vi "Acquisition_Dialog.vi"(1 "Scan Parameters file path":path, 11 "error in":errorcluster) -> (3 "Replay settings out":T17={"Sampling Rate"=0.0, "Samples in replay"=0, "Replay Start Time"=1000.0, "Replay Stop Time"=0.003} {"Replay Stop Time" format="%.3p"; "Replay Start Time" format="%.3p"}, 4 "Acquisition Unit Out":i32, 6 "Acquire Defn Out":T1={"Acquire Mode"=enum."stop", "Acquisition mode"=enum."Sampled", "Acquirer"=enum."Cleverscope", "Transfer Chans"=enum."Chan A+B", "A max scale"=5.0, "A min scale"=-5.0, "B max scale"=5.0, "B min scale"=-5.0, "A Probe"=enum."x1", "B Probe"=enum."x1", "A Coupling"=enum."DC", "B Coupling"=enum."DC", "A Bandwidth"=1, "B Bandwidth"=1, "Trigger Source"=enum."Chan A", "Trigger Amplitude"=0.0, "A Trigger Amplitude"=0.0, "B Trigger Amplitude"=0.0, "Trigger Filter"=enum."None", "Trig Slope"=FALSE, "Trigger Holdoff"=0.0, "Dig Pattern Rqd"=FALSE, "Dig Pattern"=0, "Ext Trig Threshold"=0.0, "Dig Input Threshold"=0.0, "Start Time"=-0.003, "Stop Time"=0.003, "Pre Trig Time"=0.003, "Port"=enum."Port 1", "Num divisions"=6, "Num seq frames"=1, "Num Buffers"=2, "Sig Gen Freq"=1000.0, "Sig Gen Amp"=1.0, "Sig Gen Offset"=0.0, "Sig Gen Waveform"=enum."sine", "Sig Gen Sweep"=enum."Log", "Sig Gen Func"=enum."Standard", "Sig Gen Freq 2"=1000.0, "Sig Gen Phase"=180.0, "Trig 2 Function"=enum."None", "Min Trigger Period"=1e-08, "Max trigger Period"=0.0001, "Trigger count"=1, "Trig 2 Slope"=FALSE, "Trig 2 Source Chan"=enum."Chan A", "Trig 2 Level"=0.0, "Dig Pattern 2 Rqd"=FALSE, "Dig Pattern 2"=0, "Trigger 2 Source"=enum."Trigger 1 inverted", "Waveform Averages"=0, "Value changed"=0, "Freq Span"=0.0, "Freq Res"=0.0, "Duration"=0.0, "Resolution"=0.0, "Link Port"=enum."Debug", "Ext Sample Clock"=FALSE, "F Spare 2"=FALSE, "F Spare 3"=FALSE, "F Spare 4"=FALSE, "Sampler Resolution"=enum."10 bit", "Intf Source"=enum."USB", "Update Rate"=enum."20 Frame/sec", "Transfer Size"=enum."Normal", "Sig Gen Freq Step"=0.0, "TCP Adr"=0, "TCP port"=0, "CAU Ser Num Hi"=0, "CAU Ser Num Lo"=0, "Function Number"=0.0, "Function Parameter"=0.0, "Function Result"=0.0, "Link Start"=0, "Link Timebase"=0, "Link Timer"=0, "Link Setup"=0, "Spare 1"=0.0, "Spare 2"=0.0, "Spare 3"=0.0, "Spare 4"=0.0} {"Function Result" format="%#.6p"; "Function Parameter" format="%#.6p"; "Function Number" format="%#.6p"; "TCP Adr" format="%08x"; "Sig Gen Freq Step" format="%.2f"; "Sig Gen Phase" format="%.2f"; "Sig Gen Freq 2" format="%.2f"; "Resolution" format="%#.6p"; "Duration" format="%#.6p"; "Freq Res" format="%#.6p"; "Freq Span" format="%#.6p"; "Dig Pattern 2" format="%.0x"; "Trig 2 Level" step=0.001 format="%#.6p"; "Trigger count" step=1; "Max trigger Period" min=1e-08 max=42.9 step=0.01 format="%#.6p"; "Min Trigger Period" min=1e-08 max=42.9 step=0.01 format="%#_6p"; "Sig Gen Offset" format="%.2f"; "Sig Gen Amp" format="%.2f"; "Sig Gen Freq" format="%.2f"; "B Trigger Amplitude" format="%.1p"; "A Trigger Amplitude" format="%.1p"; "B Bandwidth" format="%x"; "A Bandwidth" format="%x"; "B min scale" format="%.2p"; "B max scale" format="%.2p"; "A min scale" format="%.2p"; "A max scale" format="%.2p"; "Trigger Holdoff" format="%.1p"; "Dig Input Threshold" format="%.2f"; "Ext Trig Threshold" format="%.2f"; "Dig Pattern" format="%.0x"; "Pre Trig Time" format="%.3p"; "Start Time" format="%.2p"; "Trigger Amplitude" format="%.1p"; "Stop Time" format="%.2p"}, 8 "Cancelled?":bool, 15 "error out":errorcluster)   [LabVIEW 2009]
uses:
  libraries/Cscope control driver.llb/Acquire Event type.ctl
  libraries/Cscope control driver.llb/Acquire capture type.ctl
  libraries/Cscope control driver.llb/Acquire capture method.ctl
  libraries/Cscope control driver.llb/Acquirer type.ctl
  libraries/Cscope control driver.llb/Input Range.ctl
  libraries/Cscope control driver.llb/Input Coupling.ctl
  libraries/Cscope control driver.llb/Input Bandwidth.ctl
  libraries/Cscope control driver.llb/USB channel.ctl
  libraries/Cscope control driver.llb/Trigger Filter.ctl
  libraries/Cscope control driver.llb/Cscope waveform type.ctl
  libraries/Cscope control driver.llb/Trigger Period.ctl
  libraries/Cscope control driver.llb/Trigger channel.ctl
  libraries/Cscope control driver.llb/Link port types.ctl
  libraries/Cscope control driver.llb/Acquirer resolution.ctl
  libraries/Cscope control driver.llb/Intf source.ctl
  libraries/Cscope control driver.llb/Acquire transfer size.ctl
  typedefs/Cscope/ReplaySettings.ctl
  libraries/Cscope control driver.llb/Digital Pattern.ctl
  libraries/Cscope control driver.llb/Digital And Or.ctl
  libraries/Cscope control driver.llb/Digital And Or option.ctl
  libraries/Cscope control driver.llb/Digital Masks.ctl
  libraries/Cscope control driver.llb/Dig Control.ctl
  typedefs/Cscope/Connection Settings.ctl
  typedefs/Cscope/TriggerDefn.ctl
  typedefs/AcquisitionDialog_States.ctl
panel:
  in  "Acquire Defn":T1={"Acquire Mode"=enum."stop", "Acquisition mode"=enum."Sampled", "Acquirer"=enum."Cleverscope", "Transfer Chans"=enum."Chan A+B", "A max scale"=5.0, "A min scale"=-5.0, "B max scale"=5.0, "B min scale"=-5.0, "A Probe"=enum."x1", "B Probe"=enum."x1", "A Coupling"=enum."DC", "B Coupling"=enum."DC", "A Bandwidth"=1, "B Bandwidth"=1, "Trigger Source"=enum."Chan A", "Trigger Amplitude"=0.0, "A Trigger Amplitude"=0.0, "B Trigger Amplitude"=0.0, "Trigger Filter"=enum."None", "Trig Slope"=FALSE, "Trigger Holdoff"=0.0, "Dig Pattern Rqd"=FALSE, "Dig Pattern"=0, "Ext Trig Threshold"=0.0, "Dig Input Threshold"=0.0, "Start Time"=-0.003, "Stop Time"=0.003, "Pre Trig Time"=0.003, "Port"=enum."Port 1", "Num divisions"=6, "Num seq frames"=1, "Num Buffers"=2, "Sig Gen Freq"=1000.0, "Sig Gen Amp"=1.0, "Sig Gen Offset"=0.0, "Sig Gen Waveform"=enum."sine", "Sig Gen Sweep"=enum."Log", "Sig Gen Func"=enum."Standard", "Sig Gen Freq 2"=1000.0, "Sig Gen Phase"=180.0, "Trig 2 Function"=enum."None", "Min Trigger Period"=1e-08, "Max trigger Period"=0.0001, "Trigger count"=1, "Trig 2 Slope"=FALSE, "Trig 2 Source Chan"=enum."Chan A", "Trig 2 Level"=0.0, "Dig Pattern 2 Rqd"=FALSE, "Dig Pattern 2"=0, "Trigger 2 Source"=enum."Trigger 1 inverted", "Waveform Averages"=0, "Value changed"=0, "Freq Span"=0.0, "Freq Res"=0.0, "Duration"=0.0, "Resolution"=0.0, "Link Port"=enum."Debug", "Ext Sample Clock"=FALSE, "F Spare 2"=FALSE, "F Spare 3"=FALSE, "F Spare 4"=FALSE, "Sampler Resolution"=enum."10 bit", "Intf Source"=enum."USB", "Update Rate"=enum."20 Frame/sec", "Transfer Size"=enum."Normal", "Sig Gen Freq Step"=0.0, "TCP Adr"=0, "TCP port"=0, "CAU Ser Num Hi"=0, "CAU Ser Num Lo"=0, "Function Number"=0.0, "Function Parameter"=0.0, "Function Result"=0.0, "Link Start"=0, "Link Timebase"=0, "Link Timer"=0, "Link Setup"=0, "Spare 1"=0.0, "Spare 2"=0.0, "Spare 3"=0.0, "Spare 4"=0.0} {"Function Result" format="%#.6p"; "Function Parameter" format="%#.6p"; "Function Number" format="%#.6p"; "TCP Adr" format="%08x"; "Sig Gen Freq Step" format="%.2f"; "Sig Gen Phase" format="%.2f"; "Sig Gen Freq 2" format="%.2f"; "Resolution" format="%#.6p"; "Duration" format="%#.6p"; "Freq Res" format="%#.6p"; "Freq Span" format="%#.6p"; "Dig Pattern 2" format="%.0x"; "Trig 2 Level" step=0.001 format="%#.6p"; "Trigger count" step=1; "Max trigger Period" min=1e-08 max=42.9 step=0.01 format="%#.6p"; "Min Trigger Period" min=1e-08 max=42.9 step=0.01 format="%#_6p"; "Sig Gen Offset" format="%.2f"; "Sig Gen Amp" format="%.2f"; "Sig Gen Freq" format="%.2f"; "B Trigger Amplitude" format="%.1p"; "A Trigger Amplitude" format="%.1p"; "B Bandwidth" format="%x"; "A Bandwidth" format="%x"; "B min scale" format="%.2p"; "B max scale" format="%.2p"; "A min scale" format="%.2p"; "A max scale" format="%.2p"; "Trigger Holdoff" format="%.1p"; "Dig Input Threshold" format="%.2f"; "Ext Trig Threshold" format="%.2f"; "Dig Pattern" format="%.0x"; "Pre Trig Time" format="%.3p"; "Start Time" format="%.2p"; "Trigger Amplitude" format="%.1p"; "Stop Time" format="%.2p"}
  in  "Tab Control":T18(tab)
  in  "Trigger 1 Definition":T24={"Source"=enum."Chan A", "Level"=0.0, "Slope"=FALSE, "Dig Pattern"={"Digital Or Mask"={"1"=FALSE, "2"=FALSE, "3"=FALSE, "4"=FALSE, "5"=FALSE, "6"=FALSE, "7"=FALSE, "8"=FALSE}, "Digital Masks"={"8"=enum."C", "7"=enum."C", "6"=enum."C", "5"=enum."C", "4"=enum."C", "3"=enum."C", "2"=enum."C", "1"=enum."Ý"}}, "Digital \nPattern"=FALSE, "Filter"=enum."None"} {"Level" step=0.001 format="%#.6p"}
  in  "Channel Settings":T25={"A max scale"=1.0, "A min scale"=-1.0, "B max scale"=5.0, "B min scale"=-5.0, "A Probe"=enum."x1", "B Probe"=enum."x1", "A Coupling"=enum."DC", "B Coupling"=enum."DC", "A Filter"=FALSE, "B Filter"=FALSE} {"B min scale" format="%.2p"; "B max scale" format="%.2p"; "A min scale" format="%.2p"; "A max scale" format="%.2p"}
  in  "Force Select":T26(radio)
  in  "Replay Settings":T17={"Sampling Rate"=0.0, "Samples in replay"=0, "Replay Start Time"=1000.0, "Replay Stop Time"=0.003} {"Replay Stop Time" format="%.3p"; "Replay Start Time" format="%.3p"}
  in  "Acquisition Unit":i32
  in  "Acquisition Settings":T27={"Acquire Mode"=enum."single", "Acquisition mode"=enum."Sampled", "Onboard\nWaveform Averages"=0, "Number of Averages"=1, "Sampler Resolution"=enum."12 Bit", "Ext Sample Clock"=FALSE} {"Onboard\nWaveform Averages" scale=4.0..128.0; "Number of Averages" max=2999}
  in  "Sync Signal Settings":T28={"Pulse Repitition Interval"=333.33, "Amplitude"=2.0}
  in  "Filtering":T29 {"Pre-Filter A" items=["None", "20 MHz filter"]; "Pre-Filter B" items=["None", "20 MHz filter"]; "Moving Average" items=["40 ns"=1, "80 ns"=2, "160 ns"=3, "320 ns"=4, "640 ns"=5, "1.28 us"=6]}
  in  "Trigger 2 Source":enum16{"Trigger 1 inverted", "Trig 2 Defn"}(ring)
  in  "Trigger 2 Definition":T30={"Source"=enum."Chan A", "Level"=0.0, "Slope"=FALSE, "Dig Pattern"={"Digital Or Mask"={"1"=FALSE, "2"=FALSE, "3"=FALSE, "4"=FALSE, "5"=FALSE, "6"=FALSE, "7"=FALSE, "8"=FALSE}, "Digital Masks"={"8"=enum."C", "7"=enum."C", "6"=enum."C", "5"=enum."C", "4"=enum."C", "3"=enum."C", "2"=enum."C", "1"=enum."Ý"}}, "Digital \nPattern"=FALSE} {"Level" step=0.001 format="%#.6p"}
  in  "Trig 1~2":T31={"Trig 2 Function"=enum."None", "Min Trigger Period"=1e-08, "Max trigger Period"=0.0001, "Trigger count"=1} {"Trigger count" step=1; "Max trigger Period" min=1e-08 max=42.9 step=0.01 format="%#.6p"; "Min Trigger Period" min=1e-08 max=42.9 step=0.01 format="%#_6p"}
  in  "Connection Settings":T32
  in  "Cancel":bool
  in  "OK":bool
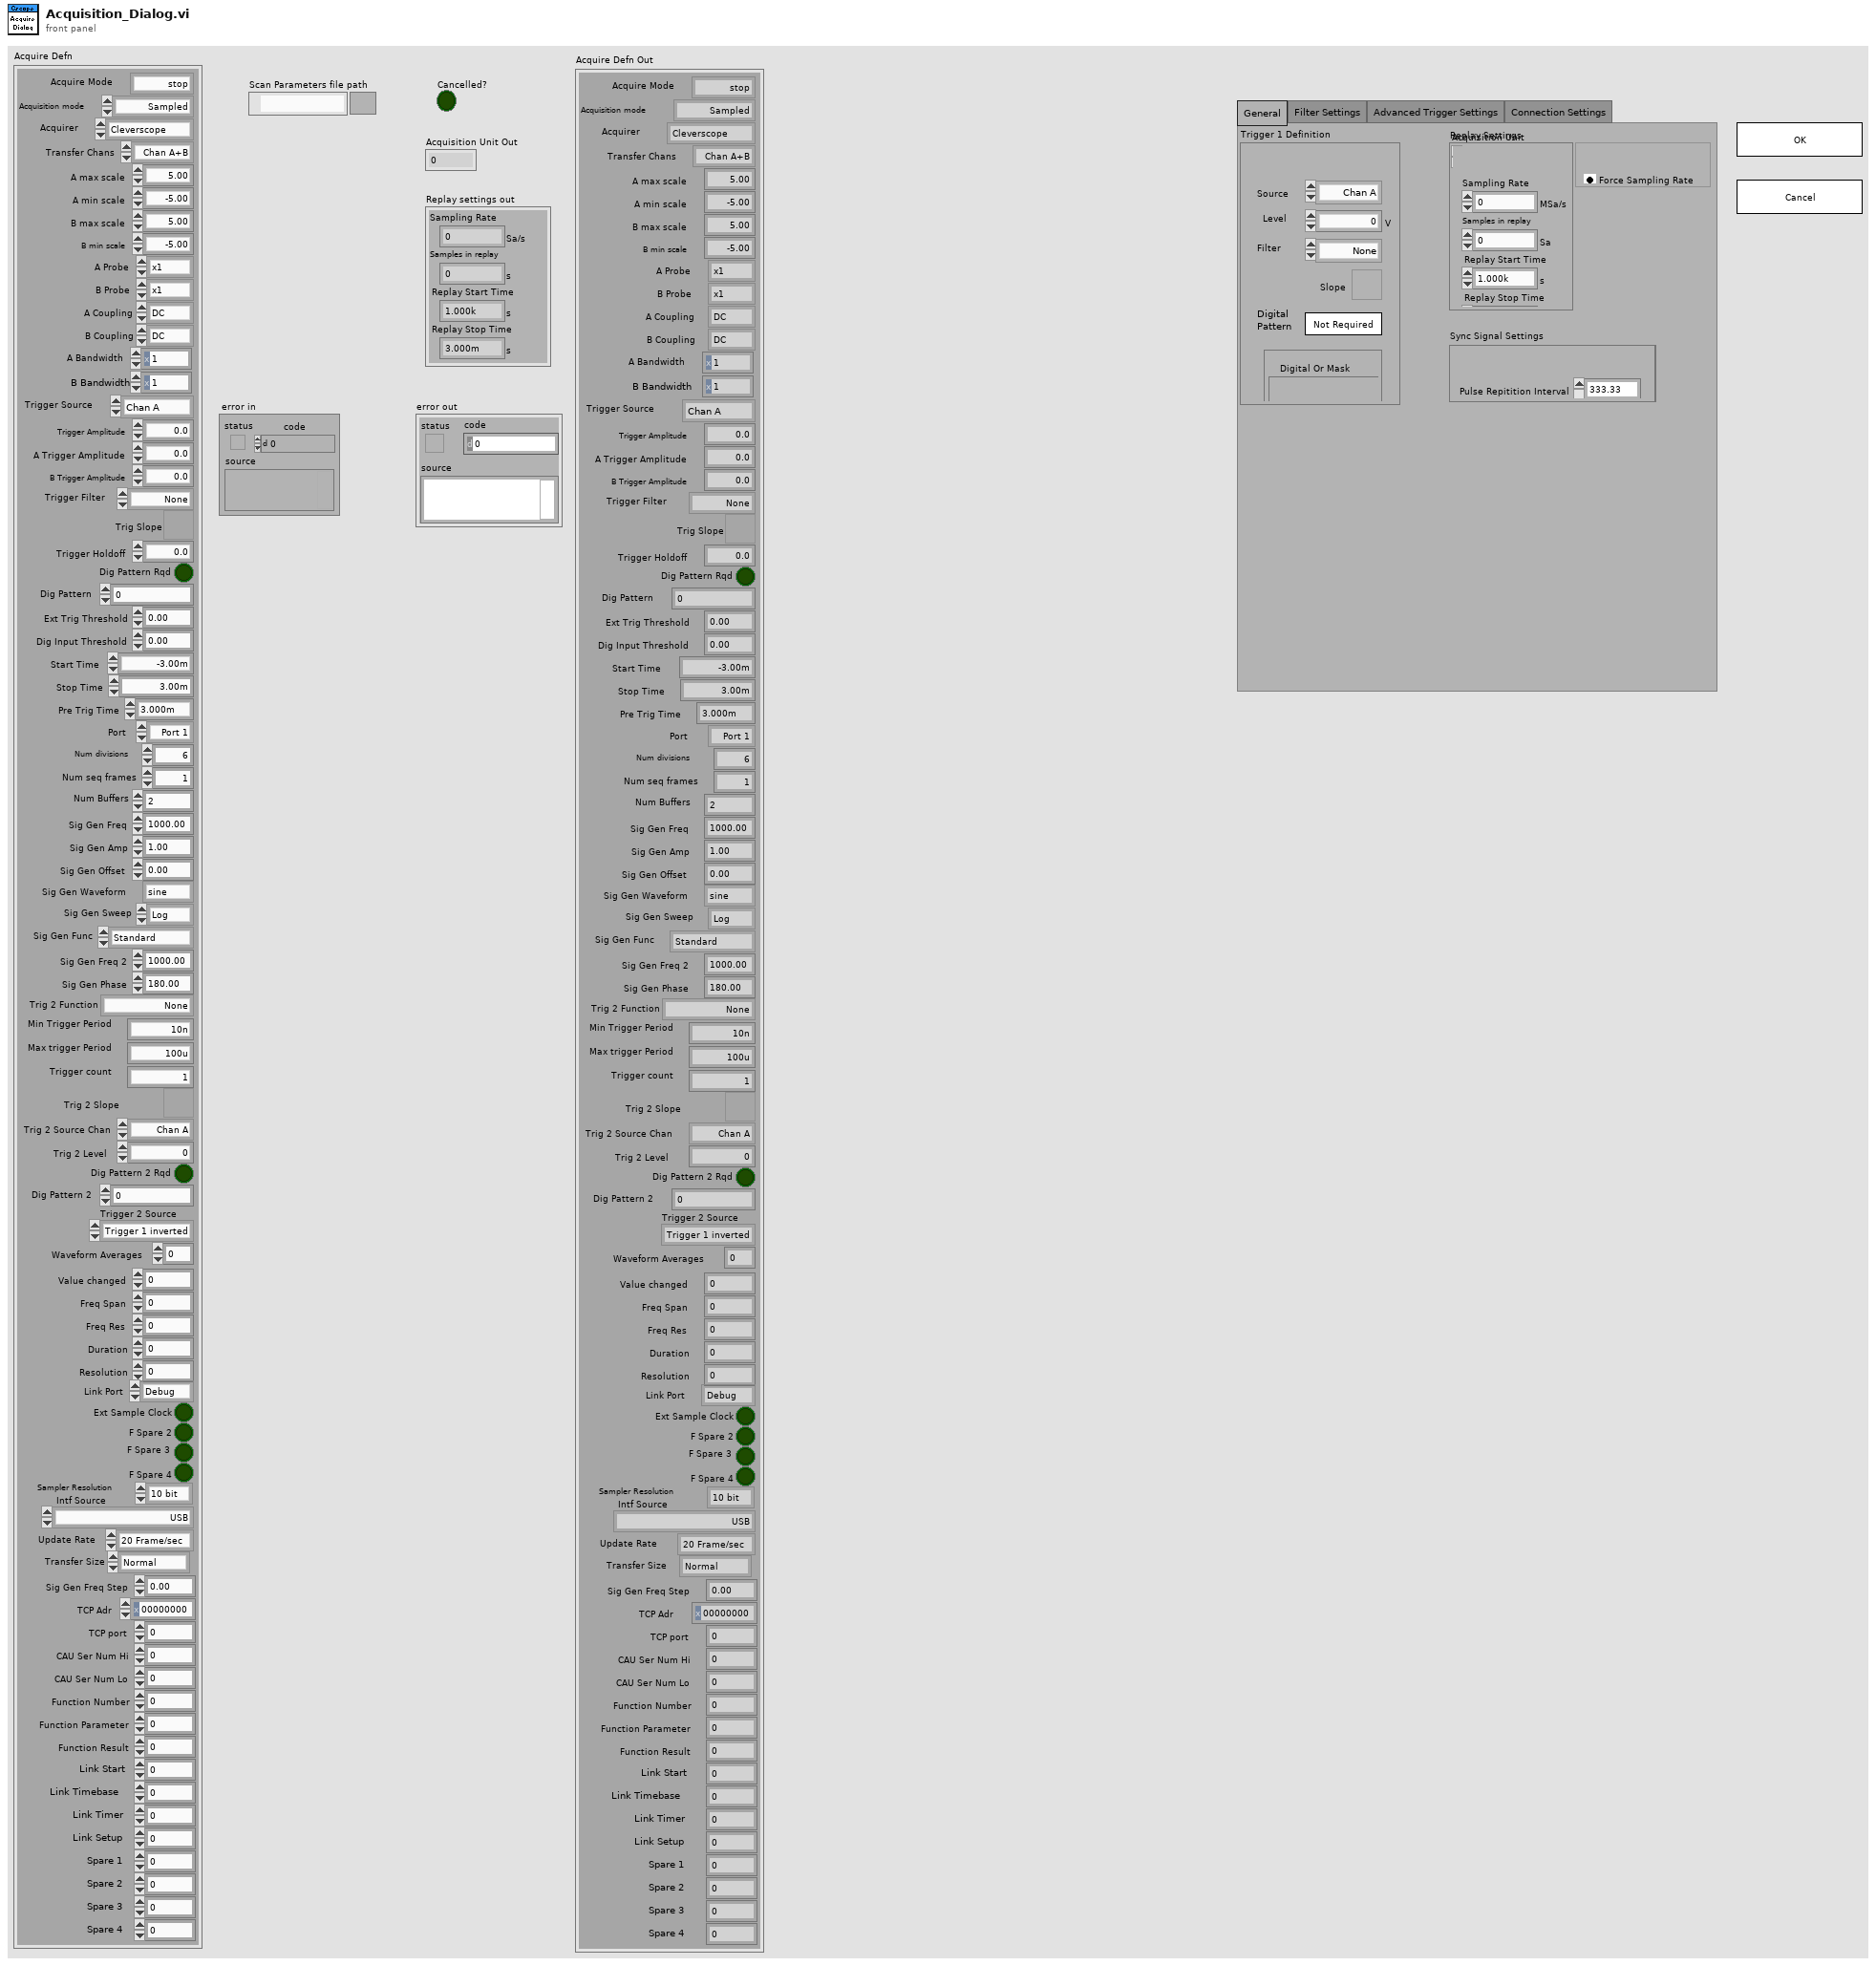
[diagram p1: front panel]
types:
  T1 = typedef "Acquire Event type.ctl" = cluster{"Acquire Mode":T2, "Acquisition mode":T3, "Acquirer":T4, "Transfer Chans":enum16{"Chan A", "Chan B", "Chan A+B"}, "A max scale":dbl, "A min scale":dbl, "B max scale":dbl, "B min scale":dbl, "A Probe":T5, "B Probe":T5, "A Coupling":T6, "B Coupling":T6, "A Bandwidth":T7, "B Bandwidth":T7, "Trigger Source":T8, "Trigger Amplitude":dbl, "A Trigger Amplitude":dbl, "B Trigger Amplitude":dbl, "Trigger Filter":T9, "Trig Slope":bool, "Trigger Holdoff":dbl, "Dig Pattern Rqd":bool, "Dig Pattern":u32, "Ext Trig Threshold":dbl, "Dig Input Threshold":dbl, "Start Time":dbl, "Stop Time":dbl, "Pre Trig Time":dbl, "Port":enum16{"Port 1", "Port 2", "Port 3", "Port 4", "Port 5", "Port 6"}, "Num divisions":i16, "Num seq frames":i16, "Num Buffers":i32, "Sig Gen Freq":dbl, "Sig Gen Amp":dbl, "Sig Gen Offset":dbl, "Sig Gen Waveform":T10, "Sig Gen Sweep":enum16{"Linear", "Log"}, "Sig Gen Func":enum16{"Standard", "Auto advance", "Freq mod In8", "Phase mod In8"}, "Sig Gen Freq 2":dbl, "Sig Gen Phase":dbl, "Trig 2 Function":T11, "Min Trigger Period":dbl, "Max trigger Period":dbl, "Trigger count":u32, "Trig 2 Slope":bool, "Trig 2 Source Chan":T12, "Trig 2 Level":dbl, "Dig Pattern 2 Rqd":bool, "Dig Pattern 2":u32, "Trigger 2 Source":enum16{"Trigger 1 inverted", "Trig 2 Defn"}, "Waveform Averages":i32, "Value changed":i32, "Freq Span":dbl, "Freq Res":dbl, "Duration":dbl, "Resolution":dbl, "Link Port":T13, "Ext Sample Clock":bool, "F Spare 2":bool, "F Spare 3":bool, "F Spare 4":bool, "Sampler Resolution":T14, "Intf Source":T15, "Update Rate":enum16{"20 Frame/sec", "10 Frame/sec", "5 Frame/sec"}, "Transfer Size":T16, "Sig Gen Freq Step":dbl, "TCP Adr":u32, "TCP port":u32, "CAU Ser Num Hi":u32, "CAU Ser Num Lo":u32, "Function Number":dbl, "Function Parameter":dbl, "Function Result":dbl, "Link Start":u32, "Link Timebase":u32, "Link Timer":u32, "Link Setup":u32, "Spare 1":dbl, "Spare 2":dbl, "Spare 3":dbl, "Spare 4":dbl}
  T2 = typedef "Acquire capture type.ctl" = enum16{"single", "automatic", "triggered", "stop", "single stop", "replay"}
  T3 = typedef "Acquire capture method.ctl" = enum16{"Sampled", "Peak Captured", "Filtered", "Repetitive", "Waveform avg"}
  T4 = typedef "Acquirer type.ctl" = enum16{"Internal Sig Gen", "APC 901", "APC 901A", "Sound Card", "Cleverscope"}
  T5 = typedef "Input Range.ctl" = enum16{"x1", "x10", "x100", "x1K", "x20", "x50", "x200"}
  T6 = typedef "Input Coupling.ctl" = enum16{"AC", "DC"}
  T7 = typedef "Input Bandwidth.ctl" = u16
  T8 = typedef "USB channel.ctl" = enum32{"Chan A", "Chan B", "Ext Trigger", "Dig Trig", "Link Input", "chan_5", "chan_6", "chan_7", "chan_8", "chan_9", "chan_10", "chan_11", "chan_12", "chan_13", "chan_14", "chan_15"}
  T9 = typedef "Trigger Filter.ctl" = enum16{"None", "Low Pass", "Hi Pass", "Noise"}
  T10 = typedef "Cscope waveform type.ctl" = enum16{"sine", "triangle", "square", "DC", "OFF"}
  T11 = typedef "Trigger Period.ctl" = enum16{"None", "Trig 1~2 < min", "min<T1~2 < max", "Trig 1~2 > max", "Count Trig 1", "Count Trig 2"}
  T12 = typedef "Trigger channel.ctl" = enum32{"Chan A", "Chan B", "Ext Trigger", "Dig Trig", "Link Input"}
  T13 = typedef "Link port types.ctl" = enum8{"Debug", "Link Out", "Disabled", "Slave", "Master", "Uart", "SPI", "I2C", "Digital", "Sig Gen"}
  T14 = typedef "Acquirer resolution.ctl" = enum16{"10 bit", "12 Bit", "14 bit"}
  T15 = typedef "Intf source.ctl" = enum16{"USB", "Ethernet - Find by IP address", "Ethernet - Find first IP address", "Ethernet - Find by serial number"}
  T16 = typedef "Acquire transfer size.ctl" = enum16{"Normal", "100% Buffer", "50% Buffer", "10% Buffer", "5% Buffer", "2% Buffer", "Sequence"}
  T17 = typedef "ReplaySettings.ctl" = cluster{"Sampling Rate":dbl, "Samples in replay":u32, "Replay Start Time":dbl, "Replay Stop Time":dbl}
  T18 = enum32{"General", "Filter Settings", "Advanced Trigger Settings", "Connection Settings"}
  T19 = typedef "Digital Pattern.ctl" = cluster{"Digital Or Mask":T20, "Digital Masks":T22}
  T20 = typedef "Digital And Or.ctl" = cluster{"1":T21, "2":T21, "3":T21, "4":T21, "5":T21, "6":T21, "7":T21, "8":T21}
  T21 = typedef "Digital And Or option.ctl" = bool
  T22 = typedef "Digital Masks.ctl" = cluster{"8":T23, "7":T23, "6":T23, "5":T23, "4":T23, "3":T23, "2":T23, "1":T23}
  T23 = typedef "Dig Control.ctl" = enum16{"0", "1", "C", "Ý", "ß"}
  T24 = cluster{"Source":T12, "Level":dbl, "Slope":bool, "Dig Pattern":T19, "Digital \nPattern":bool, "Filter":T9}
  T25 = cluster{"A max scale":dbl, "A min scale":dbl, "B max scale":dbl, "B min scale":dbl, "A Probe":T5, "B Probe":T5, "A Coupling":T6, "B Coupling":T6, "A Filter":bool, "B Filter":bool}
  T26 = enum32{"Force Sampling Rate", "Force Sample Count"}
  T27 = cluster{"Acquire Mode":T2, "Acquisition mode":T3, "Onboard\nWaveform Averages":u8, "Number of Averages":u16, "Sampler Resolution":T14, "Ext Sample Clock":bool}
  T28 = cluster{"Pulse Repitition Interval":dbl, "Amplitude":dbl}
  T29 = cluster{"Pre-Filter A":u8, "Pre-Filter B":u8, "Moving Average":u8, "Moving Average A":bool, "Moving Average B":bool}
  T30 = typedef "TriggerDefn.ctl" = cluster{"Source":T12, "Level":dbl, "Slope":bool, "Dig Pattern":T19, "Digital \nPattern":bool}
  T31 = cluster{"Trig 2 Function":T11, "Min Trigger Period":dbl, "Max trigger Period":dbl, "Trigger count":u32}
  T32 = typedef "Connection Settings.ctl" = cluster{"Intf Source":T15, "TCP Address":string, "TCP port":u32, "Serial Number":string}
  T33 = typedef "AcquisitionDialog_States.ctl" = enum16{"Handle FP Event", "Exit", "Initialize", "Force Select", "Read Parameters", "Write Parameters"}
  T34 = enum16{"Standard", "Auto advance", "Freq mod In8", "Phase mod In8"}
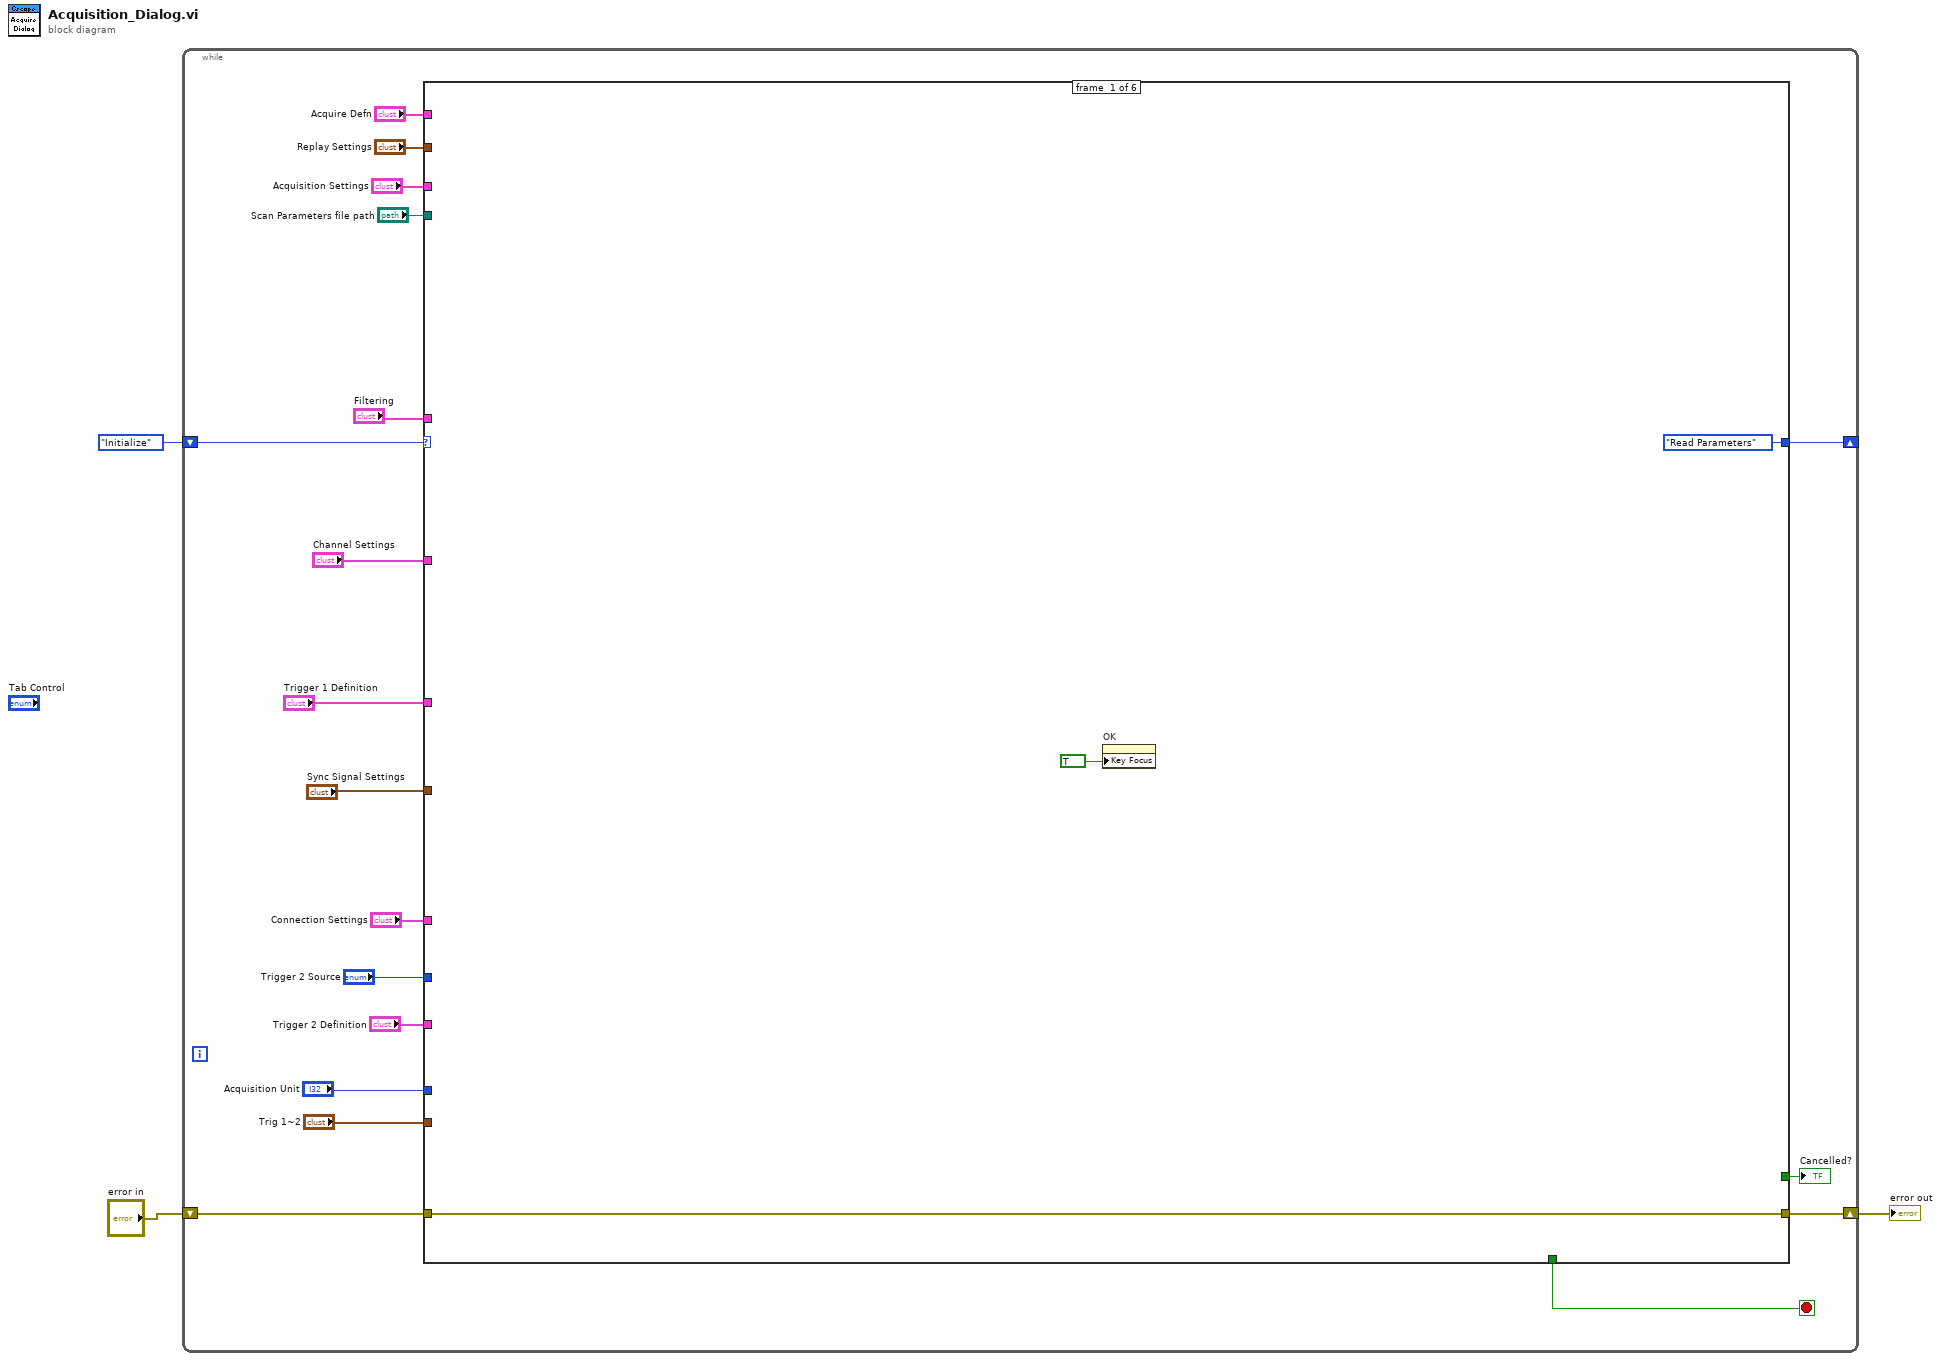
[diagram p0: block diagram]
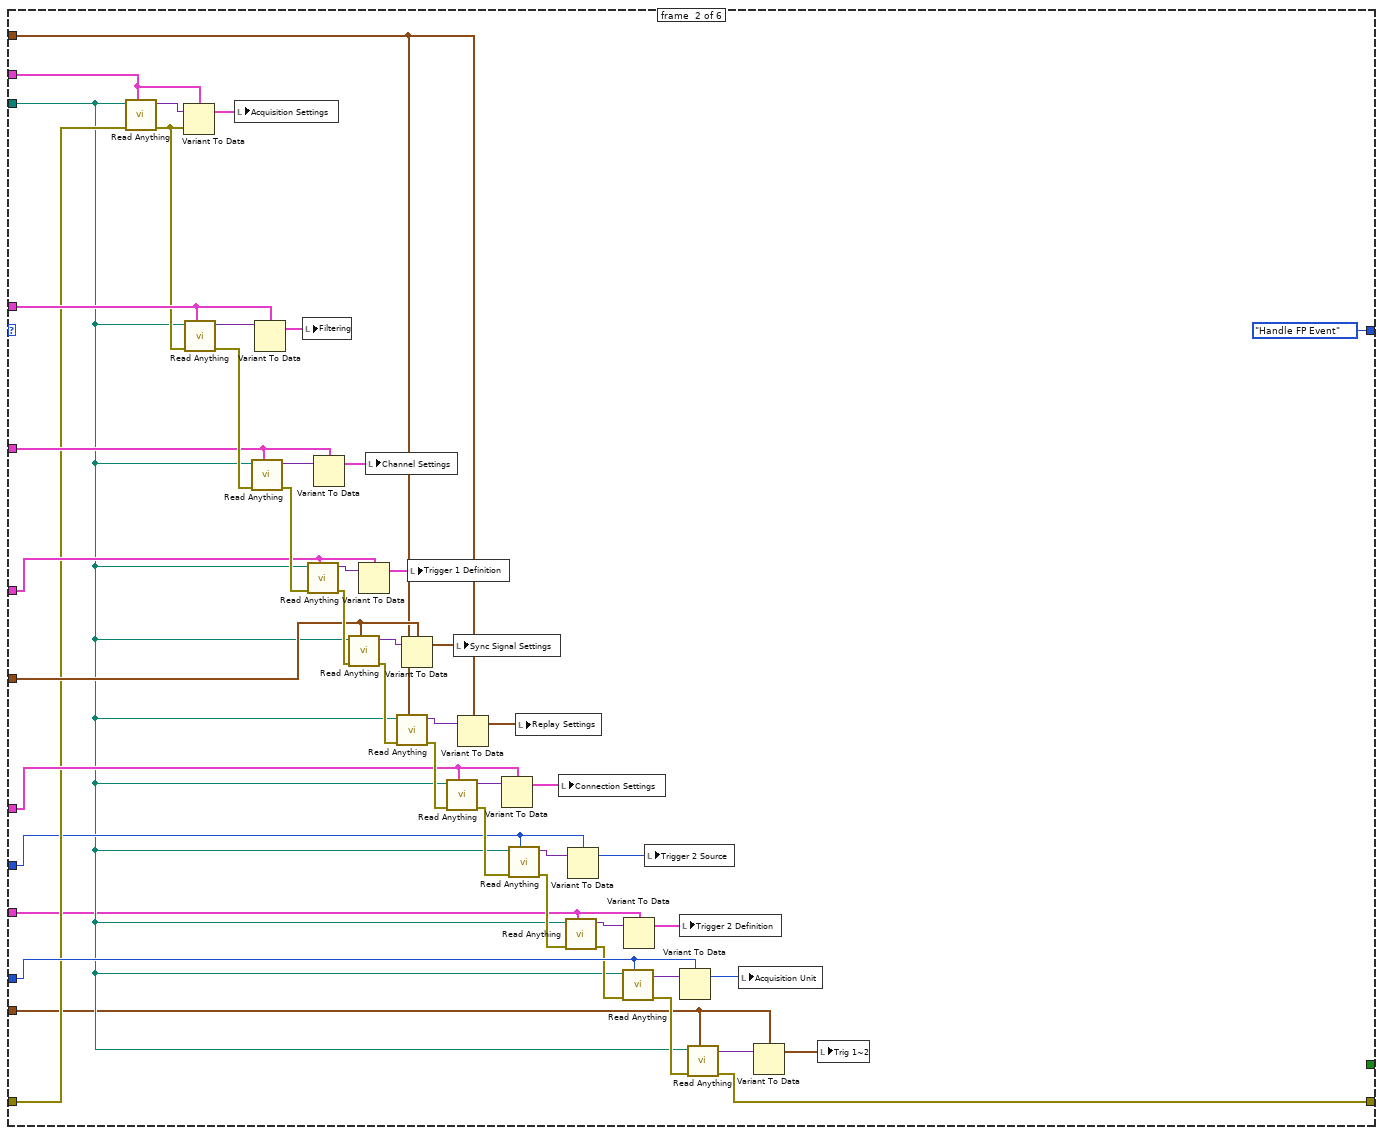
[diagram p2: hidden frame]
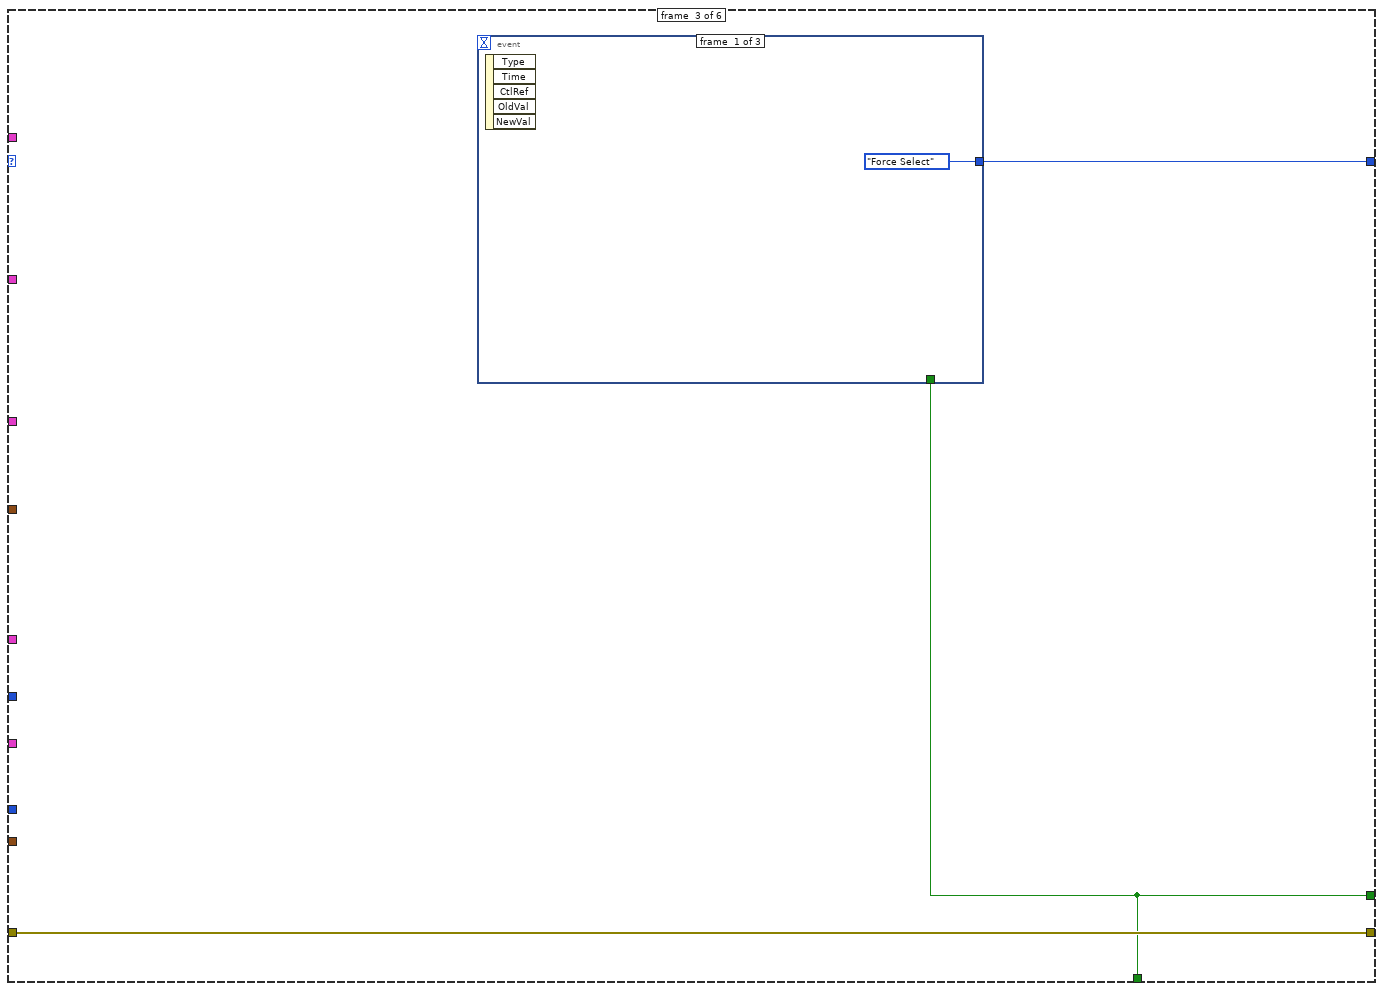
[diagram p3: hidden frame]
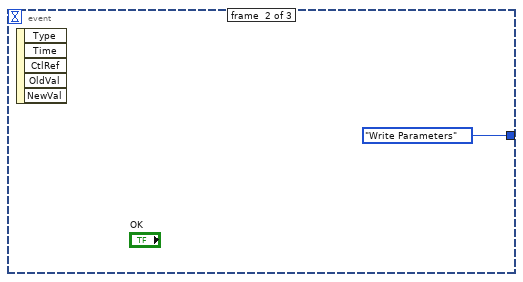
[diagram p4: hidden frame]
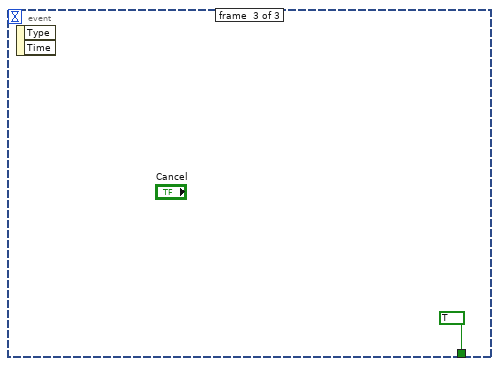
[diagram p5: hidden frame]
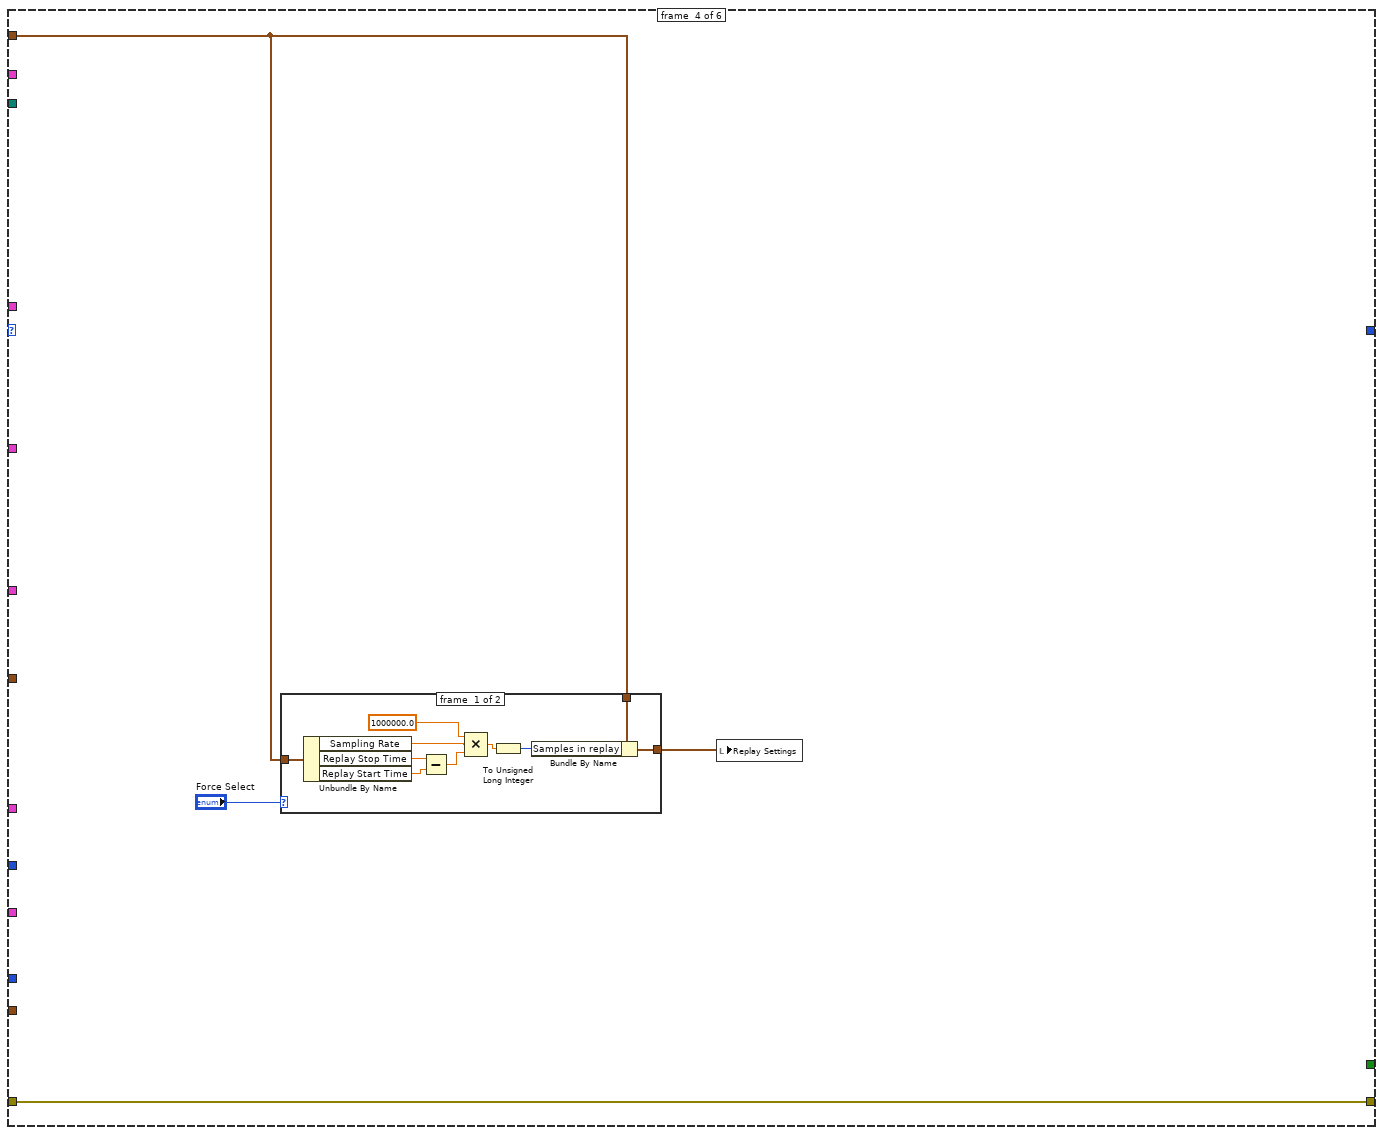
[diagram p6: hidden frame]
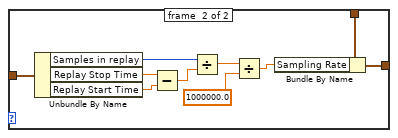
[diagram p7: hidden frame]
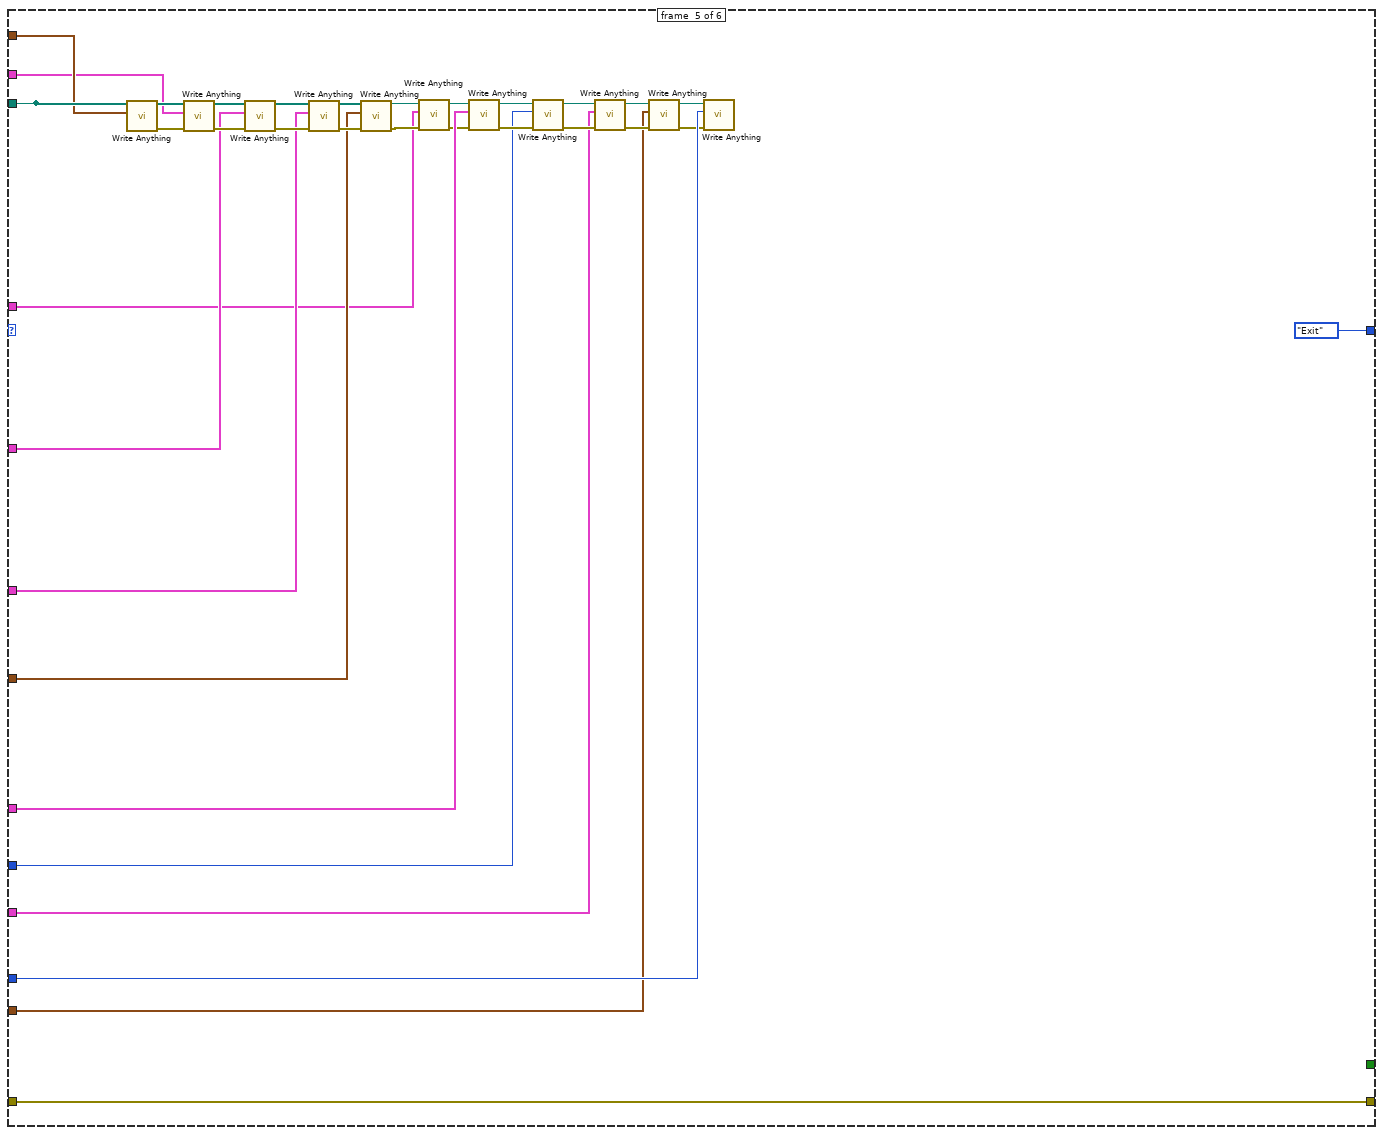
[diagram p8: hidden frame]
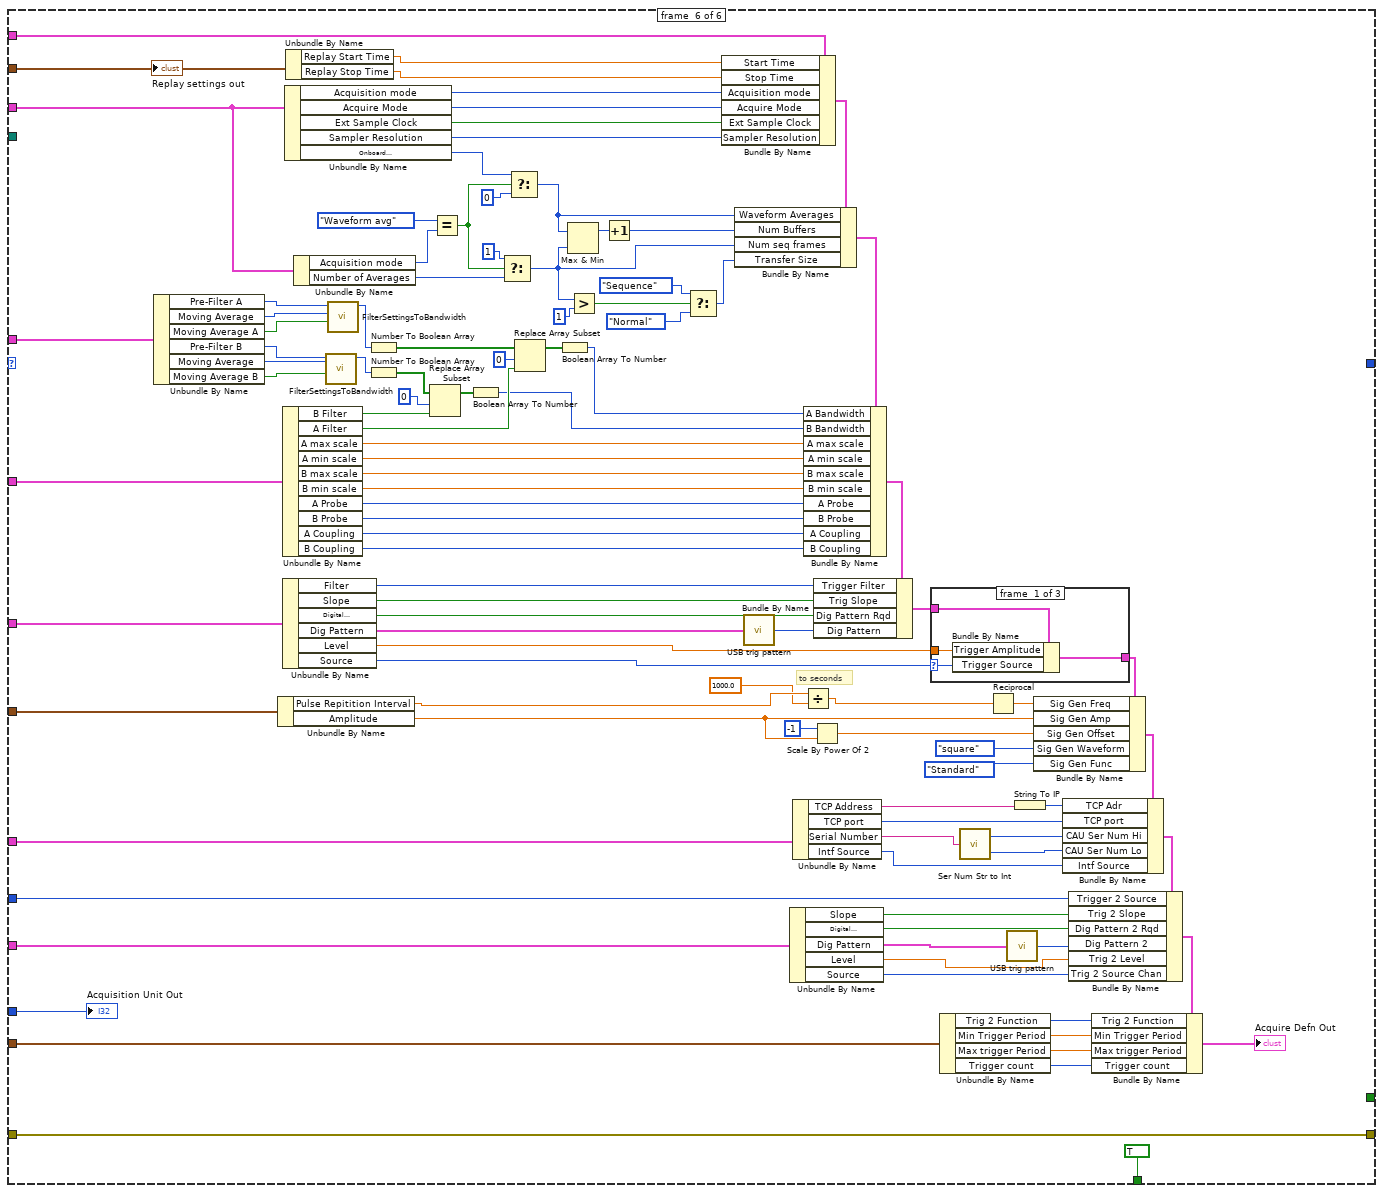
[diagram p9: hidden frame]
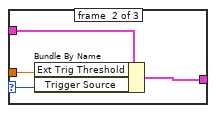
[diagram p10: hidden frame]
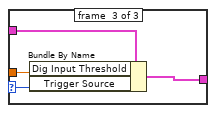
[diagram p11: hidden frame]
diagram:
  n1 = while {
    shift-right: [w21] -> w1
    shift-left: "error in" -> [w22]
    shift-right: [w15] -> _
    shift-left: AcquisitionDialog_States."Initialize" -> [w19]
    stop <- w17 stop-if-true
    n2 = case shown="\"Exit\"" w19 {
      tunnel: w22 -> [w23 w38 w75 w82 w126 w137]
      tunnel: [w23 w33 w75 w82 w126 w137] -> w21
      tunnel: "Replay Settings" -> [_ w52 _ w80 w106 w135]
      tunnel: "Acquire Defn" -> [_ _ _ _ _ w174]
      tunnel: [_ _ w73 _ _ TRUE] -> w17
      tunnel: [_ _ w73 _ _ _] -> w16
      tunnel: [AcquisitionDialog_States."Read Parameters" AcquisitionDialog_States."Handle FP Event" w74 _ AcquisitionDialog_States."Exit" _] -> w15
      tunnel: "Scan Parameters file path" -> [_ w32 _ _ w109 _]
      tunnel: "Acquisition Settings" -> [_ w71 _ _ w105 w144]
      tunnel: "Filtering" -> [_ w68 _ _ w104 w143]
      tunnel: "Channel Settings" -> [_ w63 _ _ w122 w142]
      tunnel: "Trigger 1 Definition" -> [_ w59 _ _ w121 w141]
      tunnel: "Sync Signal Settings" -> [_ w55 _ _ w119 w140]
      tunnel: "Connection Settings" -> [_ w46 _ _ w118 w139]
      tunnel: "Acquisition Unit" -> [_ w41 _ _ w113 w138]
      tunnel: "Trig 1~2" -> [_ w27 _ _ w107 w132]
      tunnel: "Trigger 2 Definition" -> [_ w30 _ _ w108 w131]
      tunnel: "Trigger 2 Source" -> [_ w37 _ _ w112 w130]
      frame #0 {
        n3 = property on="OK" class="Bool"("Key Focus"=TRUE) -> ()  [unwired: 2 in, 2 out]
      }
      frame #1 {
        n4 = call "Read Anything.vi"("Type of Anything"=w71, "Error In"=w38, "Path (dialog)"=w32) -> ("Error Out"=w66:errorcluster, "Anything"=w72:variant)  [unwired: 6 in, 1 out]
        n5 = Variant To Data(error in=w66, Variant=w72, type=w71) -> (data=w70:T27)  [unwired: 1 out]
        n6 = call "Read Anything.vi"("Type of Anything"=w68, "Error In"=w66, "Path (dialog)"=w32) -> ("Error Out"=w65:errorcluster, "Anything"=w69:variant)  [unwired: 6 in, 1 out]
        n7 = local write "Acquisition Settings"(w70) -> ()
        n8 = call "Read Anything.vi"("Type of Anything"=w63, "Error In"=w65, "Path (dialog)"=w32) -> ("Error Out"=w61:errorcluster, "Anything"=w64:variant)  [unwired: 6 in, 1 out]
        n9 = Variant To Data(Variant=w69, type=w68) -> (data=w67:T29)  [unwired: 1 in, 1 out]
        n10 = local write "Filtering"(w67) -> ()
        n11 = call "Read Anything.vi"("Type of Anything"=w59, "Error In"=w61, "Path (dialog)"=w32) -> ("Error Out"=w57:errorcluster, "Anything"=w60:variant)  [unwired: 6 in, 1 out]
        n12 = Variant To Data(Variant=w64, type=w63) -> (data=w62:T25)  [unwired: 1 in, 1 out]
        n13 = call "Read Anything.vi"("Type of Anything"=w55, "Error In"=w57, "Path (dialog)"=w32) -> ("Error Out"=w53:errorcluster, "Anything"=w56:variant)  [unwired: 6 in, 1 out]
        n14 = Variant To Data(Variant=w60, type=w59) -> (data=w58:T24)  [unwired: 1 in, 1 out]
        n15 = local write "Channel Settings"(w62) -> ()
        n16 = call "Read Anything.vi"("Type of Anything"=w52, "Error In"=w53, "Path (dialog)"=w32) -> ("Error Out"=w49:errorcluster, "Anything"=w51:variant)  [unwired: 6 in, 1 out]
        n17 = Variant To Data(Variant=w56, type=w55) -> (data=w54:T28)  [unwired: 1 in, 1 out]
        n18 = local write "Trigger 1 Definition"(w58) -> ()
        n19 = call "Read Anything.vi"("Type of Anything"=w46, "Error In"=w49, "Path (dialog)"=w32) -> ("Error Out"=w48:errorcluster, "Anything"=w47:variant)  [unwired: 6 in, 1 out]
        n20 = local write "Sync Signal Settings"(w54) -> ()
        n21 = Variant To Data(Variant=w51, type=w52) -> (data=w44:T17)  [unwired: 1 in, 1 out]
        n22 = Variant To Data(Variant=w47, type=w46) -> (data=w45:T32)  [unwired: 1 in, 1 out]
        n23 = call "Read Anything.vi"("Type of Anything"=w37, "Error In"=w48, "Path (dialog)"=w32) -> ("Error Out"=w36:errorcluster, "Anything"=w50:variant)  [unwired: 6 in, 1 out]
        n24 = local write "Replay Settings"(w44) -> ()
        n25 = local write "Connection Settings"(w45) -> ()
        n26 = call "Read Anything.vi"("Type of Anything"=w30, "Error In"=w36, "Path (dialog)"=w32) -> ("Error Out"=w35:errorcluster, "Anything"=w31:variant)  [unwired: 6 in, 1 out]
        n27 = Variant To Data(Variant=w50, type=w37) -> (data=w43:enum16{"Trigger 1 inverted", "Trig 2 Defn"})  [unwired: 1 in, 1 out]
        n28 = call "Read Anything.vi"("Type of Anything"=w41, "Error In"=w35, "Path (dialog)"=w32) -> ("Error Out"=w34:errorcluster, "Anything"=w42:variant)  [unwired: 6 in, 1 out]
        n29 = Variant To Data(Variant=w31, type=w30) -> (data=w29:T30)  [unwired: 1 in, 1 out]
        n30 = local write "Trigger 2 Source"(w43) -> ()
        n31 = local write "Trigger 2 Definition"(w29) -> ()
        n32 = Variant To Data(Variant=w42, type=w41) -> (data=w40:i32)  [unwired: 1 in, 1 out]
        n33 = call "Read Anything.vi"("Type of Anything"=w27, "Error In"=w34, "Path (dialog)"=w32) -> ("Error Out"=w33:errorcluster, "Anything"=w28:variant)  [unwired: 6 in, 1 out]
        n34 = local write "Acquisition Unit"(w40) -> ()
        n35 = Variant To Data(Variant=w28, type=w27) -> (data=w26:T31)  [unwired: 1 in, 1 out]
        n36 = local write "Trig 1~2"(w26) -> ()
      }
      frame #2 {
        n37 = event shown="[2] \"Cancel\": Value Change;  Panel Close" {
          selector: _ -> [_ _ _]
          dyn-events: _ -> [_ _ _]
          timeout: _ -> [_ _ _]
          tunnel: [AcquisitionDialog_States."Force Select" AcquisitionDialog_States."Write Parameters" _] -> w74
          tunnel: [_ _ TRUE ("Cancelled?")] -> w73
          event #0 {
            n38 = event-data() -> ()  [unwired: 1 in, 5 out]
          }
          event #1 {
            n39 = event-data() -> ()  [unwired: 1 in, 5 out]
          }
          event #2 {
            n40 = event-data() -> ()  [unwired: 1 in, 2 out]
          }
        }
      }
      frame #3 {
        n41 = case shown="\"Force Sample Count\"" "Force Select" {
          tunnel: w80 -> [w87 w98]
          tunnel: [w86 w97] -> w79
          tunnel: w80 -> [w85 w96]
          frame #0 {
            n42 = Unbundle By Name(w85) -> ("Sampling Rate"=w84:dbl, "Replay Stop Time"=w92:dbl, "Replay Start Time"=w91:dbl)
            n43 = Subtract(x=w92, y=w91) -> (x-y=w90:dbl)
            n44 = Compound Arithmetic op=MULTIPLY(1000000.0 ("x"), w84, w90) -> (w89:dbl)
            n45 = To Unsigned Long Integer(number=w89) -> (unsigned 32bit integer=w88:u32)
            n46 = Bundle By Name(cluster=w87, "Samples in replay"=w88) -> (w86:T17)
          }
          frame #1 {
            n47 = Unbundle By Name(w96) -> ("Samples in replay"=w101:u32, "Replay Stop Time"=w99:dbl, "Replay Start Time"=w100:dbl)
            n48 = Subtract(x=w99, y=w100) -> (x-y=w102:dbl)
            n49 = Divide(x=w101, y=w102) -> (x/y=w95:dbl)
            n50 = Divide(x=w95, y=1000000.0) -> (x/y=w94:dbl)
            n51 = Bundle By Name(cluster=w98, "Sampling Rate"=w94) -> (w97:T17)
          }
        }
        n52 = local write "Replay Settings"(w79) -> ()
      }
      frame #4 {
        n53 = call "Write Anything.vi"("Anything"=w106, "Path (dialog)"=w109) -> ("Error Out"=w125:errorcluster)  [unwired: 9 in]
        n54 = call "Write Anything.vi"("Error In"=w125, "Anything"=w105, "Path (dialog)"=w109) -> ("Error Out"=w124:errorcluster)  [unwired: 8 in]
        n55 = call "Write Anything.vi"("Error In"=w124, "Anything"=w122, "Path (dialog)"=w109) -> ("Error Out"=w123:errorcluster)  [unwired: 8 in]
        n56 = call "Write Anything.vi"("Error In"=w123, "Anything"=w121, "Path (dialog)"=w109) -> ("Error Out"=w120:errorcluster)  [unwired: 8 in]
        n57 = call "Write Anything.vi"("Error In"=w120, "Anything"=w119, "Path (dialog)"=w109) -> ("Error Out"=w116:errorcluster)  [unwired: 8 in]
        n58 = call "Write Anything.vi"("Error In"=w116, "Anything"=w104, "Path (dialog)"=w109) -> ("Error Out"=w117:errorcluster)  [unwired: 8 in]
        n59 = call "Write Anything.vi"("Error In"=w117, "Anything"=w118, "Path (dialog)"=w109) -> ("Error Out"=w115:errorcluster)  [unwired: 8 in]
        n60 = call "Write Anything.vi"("Error In"=w115, "Anything"=w112, "Path (dialog)"=w109) -> ("Error Out"=w110:errorcluster)  [unwired: 8 in]
        n61 = call "Write Anything.vi"("Error In"=w110, "Anything"=w108, "Path (dialog)"=w109) -> ("Error Out"=w111:errorcluster)  [unwired: 8 in]
        n62 = call "Write Anything.vi"("Error In"=w111, "Anything"=w107, "Path (dialog)"=w109) -> ("Error Out"=w103:errorcluster)  [unwired: 8 in]
        n63 = call "Write Anything.vi"("Error In"=w103, "Anything"=w113, "Path (dialog)"=w109) -> ()  [unwired: 8 in, 1 out]
      }
      frame #5 {
        # "to seconds"
        n64 = Unbundle By Name(w143) -> ("Pre-Filter A"=w150:u8, "Moving Average"=w149:u8, "Moving Average A"=w148:bool, "Pre-Filter B"=w145:u8, "Moving Average"=w146:u8, "Moving Average B"=w147:bool)
        n65 = Unbundle By Name(w140) -> ("Pulse Repitition Interval"=w128:dbl, "Amplitude"=w189:dbl)
        n66 = Unbundle By Name(w142) -> ("B Filter"=w181:bool, "A Filter"=w179:bool, "A max scale"=w198:dbl, "A min scale"=w197:dbl, "B max scale"=w196:dbl, "B min scale"=w195:dbl, "A Probe"=w194:T5, "B Probe"=w193:T5, "A Coupling"=w192:T6, "B Coupling"=w191:T6)
        n67 = Unbundle By Name(w141) -> ("Filter"=w229:T9, "Slope"=w228:bool, "Digital \nPattern"=w227:bool, "Dig Pattern"=w225:T19, "Level"=w222:dbl, "Source"=w223:T12)
        n68 = Unbundle By Name(w144) -> ("Acquisition mode"=w136:T3, "Acquire Mode"=w203:T2, "Ext Sample Clock"=w202:bool, "Sampler Resolution"=w201:T14, "Onboard\nWaveform Averages"=w188:u8)
        n69 = Unbundle By Name(w135) -> ("Replay Start Time"=w133:dbl, "Replay Stop Time"=w134:dbl)
        n70 = Unbundle By Name(w144) -> ("Acquisition mode"=w199:T3, "Number of Averages"=w208:u16)
        n71 = call "FilterSettingsToBandwidth.vi"("Moving Average Enable"=w147, "Moving Average Type"=w146, "Pre-Filter"=w145) -> ("Bandwidth"=w172:T7)  [unwired: 8 in]
        n72 = call "FilterSettingsToBandwidth.vi"("Moving Average Enable"=w148, "Moving Average Type"=w149, "Pre-Filter"=w150) -> ("Bandwidth"=w173:T7)  [unwired: 8 in]
        n73 = Number To Boolean Array(number=w173) -> (Boolean array=w180:bool[])
        n74 = Number To Boolean Array(number=w172) -> (Boolean array=w182:bool[])
        n75 = Replace Array Subset(array=w182, new element=w181, index=0) -> (w177:bool[])
        n76 = Equal?(x=Acquire_capture_method."Waveform avg", y=w199) -> (x = y?=w209:bool)
        n77 = Boolean Array To Number(Boolean array=w177) -> (number=w176:u32)
        n78 = Select(t=i16 1, s=w209, f=w208) -> (s? t:f=w206:u16)
        n79 = Select(t=w188, s=w209, f=u8 0) -> (s? t:f=w215:u8)
        n80 = Replace Array Subset(array=w180, new element=w179, index=0) -> (w178:bool[])
        n81 = Boolean Array To Number(Boolean array=w178) -> (number=w175:u32)
        n82 = Max & Min(x=w215, y=w206) -> (max(x,y)=w216:u16)  [unwired: 1 out]
        n83 = Greater?(x=w206, y=i16 1) -> (0:w213:bool)
        n84 = Increment(x=w216) -> (x+1=w210:u16)
        n85 = Select(t=Acquire_transfer_size."Sequence" ("Transfer Size"), s=w213, f=Acquire_transfer_size."Normal" ("Transfer Size")) -> (s? t:f=w205:T16)
        n86 = Bundle By Name(cluster=w174, "Start Time"=w133, "Stop Time"=w134, "Acquisition mode"=w136, "Acquire Mode"=w203, "Ext Sample Clock"=w202, "Sampler Resolution"=w201) -> (w204:T1)
        n87 = Bundle By Name(cluster=w204, "Waveform Averages"=w215, "Num Buffers"=w210, "Num seq frames"=w206, "Transfer Size"=w205) -> (w190:T1)
        n88 = call "USB trig pattern.vi"("Digital Pattern"=w225) -> ("Trig Pattern"=w226:u32)
        n89 = Unbundle By Name(w131) -> ("Slope"=w162:bool, "Digital \nPattern"=w161:bool, "Dig Pattern"=w160:T19, "Level"=w158:dbl, "Source"=w157:T12)
        n90 = Unbundle By Name(w139) -> ("TCP Address"=w168:string, "TCP port"=w167:u32, "Serial Number"=w166:string, "Intf Source"=w165:T15)
        n91 = Divide(x=w128, y=1000.0 ("x")) -> (x/y=w129:dbl)
        n92 = Bundle By Name(cluster=w190, "A Bandwidth"=w175, "B Bandwidth"=w176, "A max scale"=w198, "A min scale"=w197, "B max scale"=w196, "B min scale"=w195, "A Probe"=w194, "B Probe"=w193, "A Coupling"=w192, "B Coupling"=w191) -> (w185:T1)
        n93 = Scale By Power Of 2(n=i16 -1, x=w189) -> (x*2^n=w218:dbl)
        n94 = Bundle By Name(cluster=w185, "Trigger Filter"=w229, "Trig Slope"=w228, "Dig Pattern Rqd"=w227, "Dig Pattern"=w226) -> (w224:T1)
        n95 = case shown="\"Ext Trigger\"" w223 {
          selector: w223 -> [w233 w238 w242]
          tunnel: [w234 w236 w241] -> w186
          tunnel: w224 -> [w232 w237 w240]
          tunnel: w222 -> [w231 w235 w239]
          frame #0 {
            n96 = Bundle By Name(cluster=w232, "Trigger Amplitude"=w231, "Trigger Source"=w233) -> (w234:T1)
          }
          frame #1 {
            n97 = Bundle By Name(cluster=w237, "Ext Trig Threshold"=w235, "Trigger Source"=w238) -> (w236:T1)
          }
          frame #2 {
            n98 = Bundle By Name(cluster=w240, "Dig Input Threshold"=w239, "Trigger Source"=w242) -> (w241:T1)
          }
        }
        n99 = Unbundle By Name(w132) -> ("Trig 2 Function"=w155:T11, "Min Trigger Period"=w154:dbl, "Max trigger Period"=w153:dbl, "Trigger count"=w152:u32)
        n100 = call "Ser Num Str to Int.vi"("Serial Number"=w166) -> ("Ser Num Hi"=w170:u32, "Ser Num Lo"=w169:u32)
        n101 = Reciprocal(x=w129) -> (1/x=w217:dbl)
        n102 = call "USB trig pattern.vi"("Digital Pattern"=w160) -> ("Trig Pattern"=w159:u32)
        n103 = String To IP(1:w168) -> (0:w164:u32)
        n104 = Bundle By Name(cluster=w186, "Sig Gen Freq"=w217, "Sig Gen Amp"=w189, "Sig Gen Offset"=w218, "Sig Gen Waveform"=Cscope_waveform_type."square", "Sig Gen Func"=T34."Standard") -> (w171:T1)
        n105 = Bundle By Name(cluster=w171, "TCP Adr"=w164, "TCP port"=w167, "CAU Ser Num Hi"=w170, "CAU Ser Num Lo"=w169, "Intf Source"=w165) -> (w163:T1)
        n106 = Bundle By Name(cluster=w163, "Trigger 2 Source"=w130, "Trig 2 Slope"=w162, "Dig Pattern 2 Rqd"=w161, "Dig Pattern 2"=w159, "Trig 2 Level"=w158, "Trig 2 Source Chan"=w157) -> (w156:T1)
        n107 = Bundle By Name(cluster=w156, "Trig 2 Function"=w155, "Min Trigger Period"=w154, "Max trigger Period"=w153, "Trigger count"=w152) -> (→"Acquire Defn Out":T1)
        "Acquisition Unit Out" <- w138
        "Replay settings out" <- w135
      }
    }
    "Cancelled?" <- w16
  }
  "error out" <- w1
